vi "Screen Hard Copy Settings.vi"(0 "VISA resource name":refnum<visa-resource-name>, 5 "Format (0:BMP)":i32(ring) items=["BMP", "PNG"], 7 "Flag (0:Normal)":i32(ring) items=["Normal", "Reverse"], 9 "Filename (TEST)":string="TEST", 11 "error in (no error)":errorcluster, 12 "Driver Letter (D)":string="D") -> (4 "VISA resource name out":refnum<visa-resource-name>, 15 "error out":errorcluster)   [LabVIEW 2020, in "Anritsu Signal Analyzer Series.lvlib"]
doc: "Sets the screen hard copy Setting."
uses:
  Anritsu Signal Analyzer Series.lvlib
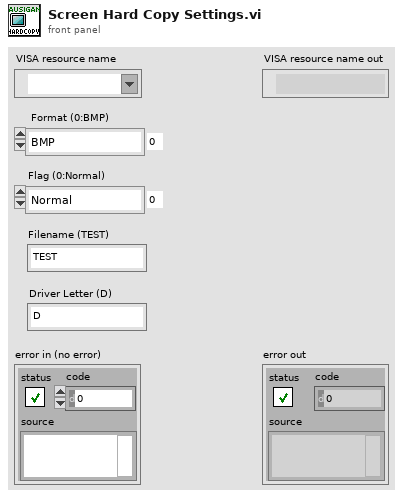
[diagram p1: front panel]
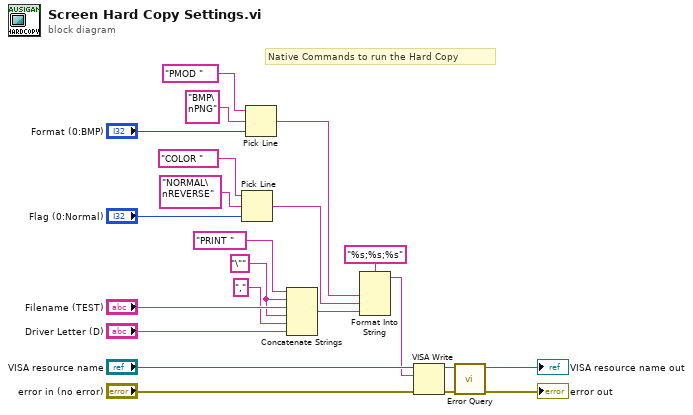
[diagram p0: block diagram]
diagram:
  w14 = "\"" ("string")
  # "Native Commands to run the Hard Copy"
  n1 = Pick Line(string ("")="COLOR " ("_Command"), multi-line string="NORMAL\nREVERSE" ("_Case0"), line index="Flag (0:Normal)") -> (output string=w1:string)
  n2 = Pick Line(string ("")="PMOD " ("_Command"), multi-line string="BMP\nPNG" ("_Case0"), line index="Format (0:BMP)") -> (output string=w4:string)
  n3 = Concatenate Strings("PRINT " ("_Command"), w14, "Filename (TEST)", w14, "," ("string"), "Driver Letter (D)") -> (w8:string)
  n4 = Format Into String(format string="%s;%s;%s" ("形式文字列"), w4, w1, w8) -> (resulting string=w7:string)  [unwired: 2 in, 1 out]
  n5 = VISA Write(VISA resource name="VISA resource name", write buffer=w7, error in (no error)="error in (no error)") -> (VISA resource name out=w11:refnum<visa-resource-name>, error out=w10:errorcluster)  [unwired: 1 out]
  n6 = call "Error Query.vi"("error in (no error)"=w10, "VISA resource name"=w11) -> ("error out"=→"error out":errorcluster, "VISA resource name out"=→"VISA resource name out":refnum<visa-resource-name>)  [unwired: 6 in, 2 out]
